vi "QueryServer_Stop.vi"(0 "Server Info":T2, 2 "Event Registration Refnum":refnum<event-registration>, 3 "error in (no error)":errorcluster) -> (10 "error out":errorcluster)   [LabVIEW 2019, in "labview-grpc-query-server.lvlib"]
uses:
  labview-grpc-query-server.lvlib
  QueryServer_InvokeEventData.ctl
  VIs/grpcId.ctl
  VIs/gprc-support.lvlib
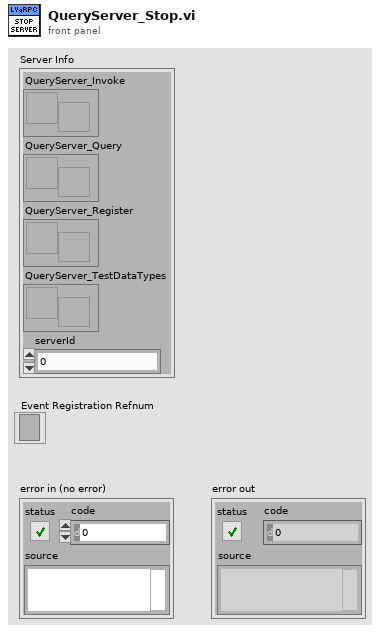
[diagram p1: front panel]
types:
  T1 = typedef "gprc-support.lvlib/grpcId.ctl" = u64
  T2 = cluster{"QueryServer_Invoke":refnum<user-event>, "QueryServer_Query":refnum<user-event>, "QueryServer_Register":refnum<user-event>, "QueryServer_TestDataTypes":refnum<user-event>, "serverId":T1}
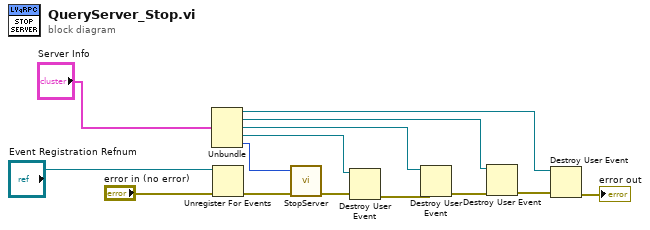
[diagram p0: block diagram]
diagram:
  n1 = Unbundle("Server Info") -> ("QueryServer_Invoke"=w8:refnum<user-event>, "QueryServer_Query"=w9:refnum<user-event>, "QueryServer_Register"=w10:refnum<user-event>, "QueryServer_TestDataTypes"=w4:refnum<user-event>, "serverId"=w1:T1)
  n2 = Unregister For Events(event registration refnum="Event Registration Refnum", error in="error in (no error)") -> (error out=w2:errorcluster)
  n3 = call "StopServer.vi"("error in (no error)"=w2, "Server Id"=w1) -> ("error out"=w3:errorcluster)  [unwired: 9 in]
  n4 = Destroy User Event(user event=w4, error in=w3) -> (error out=w5:errorcluster)
  n5 = Destroy User Event(user event=w10, error in=w5) -> (error out=w13:errorcluster)
  n6 = Destroy User Event(user event=w9, error in=w13) -> (error out=w12:errorcluster)
  n7 = Destroy User Event(user event=w8, error in=w12) -> (error out=→"error out":errorcluster)
